vi "Hierarchy To Build Order.vi"(0 "Build Analyzer in":refnum<class "Build Analyzer.lvclass">, 5 "Export Product Names to build":string[](array[string]), 7 "Build Type":T1(ring)) -> (4 "dup Build Analyzer":refnum<class "Build Analyzer.lvclass">, 6 "Ordered Exports":refnum<class "Export.lvclass">[](array[class]), 15 "error out":errorcluster)   [LabVIEW 2017, in "CL_G3_VIComponentBuilder.lvlib" / "Build Analyzer.lvclass"]
doc: "Generates the ordered set of exports to build given the product names of the exports."
uses:
  Build Analyzer.lvclass
  Exports/Exports/Export.lvclass
  Build Analyzer.lvclass/Build Analyzer.ctl
  Exports/Exports/Export.lvclass/Export.ctl
  Exports/Exports/Accessors/Read unique Name.vi
  Exports/Exports/Accessors/Read Product Name.vi
  <userlib>/_Cirrus Logic/LabVIEW Container/Source/Container/Get Child.vi
  <userlib>/_Cirrus Logic/LabVIEW Container/Source/Container/Container.lvclass
panel:
  out "Numeric":i32
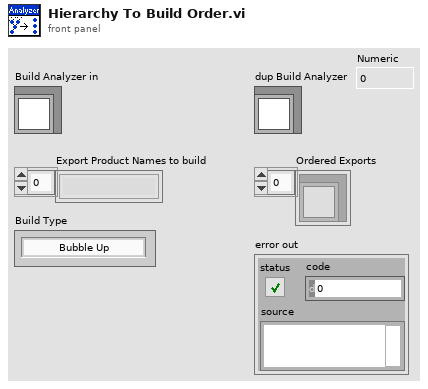
[diagram p1: front panel]
types:
  T1 = enum16{"Bubble Up", "Build Dependencies", "Build Selected Only"}
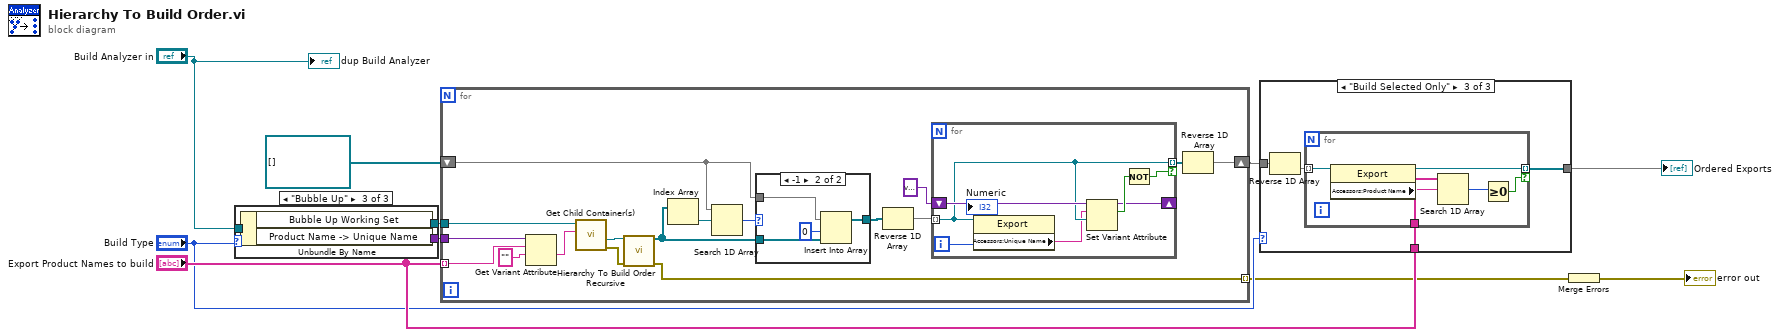
[diagram p0: block diagram]
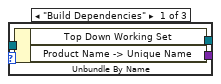
[diagram p2: hidden frame]
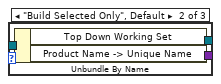
[diagram p3: hidden frame]
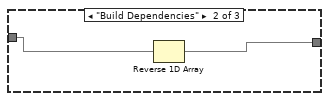
[diagram p5: hidden frame]
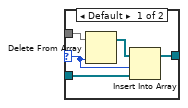
[diagram p6: hidden frame]
diagram:
  n1 = case shown="\"Bubble Up\"" "Build Type" {
    tunnel: [w13 w16 w19] -> w6
    tunnel: [w12 w15 w18] -> w4
    tunnel: "Build Analyzer in" -> [w11 w14 w17]
    frame "Build Dependencies" {
      n2 = Unbundle By Name(w11) -> ("Top Down Working Set"=w13:refnum<data-value>, "Product Name -> Unique Name"=w12:variant)
    }
    frame "Build Selected Only", Default {
      n3 = Unbundle By Name(w14) -> ("Top Down Working Set"=w16:refnum<data-value>, "Product Name -> Unique Name"=w15:variant)
    }
    frame "Bubble Up" {
      n4 = Unbundle By Name(w17) -> ("Bubble Up Working Set"=w19:refnum<data-value>, "Product Name -> Unique Name"=w18:variant)
    }
  }
  n5 = for {
    shift-right: [w20] -> w3
    shift-left: refnum<class "Export.lvclass">[] [] -> [w32]
    tunnel: w6 -> [w24]
    tunnel: "Export Product Names to build" -> [w29] mode=indexing
    tunnel: w4 -> [w30]
    tunnel: [w25] -> w7 mode=indexing
    n6 = Get Variant Attribute(Variant=w30, name=w29, default value (empty Variant)="") -> (value=w27:string)  [unwired: 1 in, 3 out]
    n7 = call-poly <userlib>:"Get Child Container(s).vi"("Container Name"=w27, "Container"=w24) -> ("error out"=w26:errorcluster, "Child Container"=w35:refnum<data-value>)  [unwired: 6 in, 2 out]
    n8 = call "Hierarchy To Build Order Recursive.vi"("Working Set"=w35, "error in (no error)"=w26) -> ("Exports"=w33:refnum<class "Export.lvclass">[], "error out"=w25:errorcluster)  [unwired: 12 in]
    n9 = Index Array(array=w33) -> (element=w34:refnum<class "Export.lvclass">)  [unwired: 1 in]
    n10 = Search 1D Array(1D array=w32, element=w34) -> (index of element=w31:i32)  [unwired: 1 in]
    n11 = case shown="-1" w31 {
      selector: w31 -> [w39 _]
      tunnel: [w37 w45] -> w23
      tunnel: w33 -> [w38 w44]
      tunnel: w32 -> [w41 w43]
      frame Default {
        n12 = Delete From Array(array=w41, index=w39) -> (array with subset deleted=w40:refnum<class "Export.lvclass">[])  [unwired: 1 in, 1 out]
        n13 = Insert Into Array(array=w40, index=w39, new element=w38) -> (w37:refnum<class "Export.lvclass">[])
      }
      frame -1 {
        n14 = Insert Into Array(array=w43, index=0, new element=w44) -> (w45:refnum<class "Export.lvclass">[])
      }
    }
    n15 = Reverse 1D Array(array=w23) -> (reversed array=w22:refnum<class "Export.lvclass">[])
    n16 = for {
      tunnel: w22 -> [w49] mode=indexing
      tunnel: [w49] -> w21 mode=indexing if=w47
      shift-right: [w50] -> _
      shift-left: variant -> [w52]
      i -> [w46]
      # "keep the"
      n17 = property class="Export"(reference=w49) -> ("Accessors:Unique Name"=w48:string)  [unwired: 1 in, 2 out]
      n18 = Set Variant Attribute(Variant=w52, name=w48, value=w49) -> (Variant out=w50:variant, replaced=w51:bool)  [unwired: 1 in, 1 out]
      n19 = Not(x=w51) -> (.not. x?=w47:bool)
      "Numeric" <- w46
    }
    n20 = Reverse 1D Array(array=w21) -> (reversed array=w20:refnum<class "Export.lvclass">[])
  }
  n21 = case shown="\"Build Selected Only\"" "Build Type" {
    tunnel: "Export Product Names to build" -> [_ _ w59]
    tunnel: [w53 w54 w58] -> w10
    tunnel: w3 -> [w53 w55 w57]
    frame "Bubble Up", Default {
    }
    frame "Build Dependencies" {
      n22 = Reverse 1D Array(array=w55) -> (reversed array=w54:refnum<class "Export.lvclass">[])
    }
    frame "Build Selected Only" {
      n23 = Reverse 1D Array(array=w57) -> (reversed array=w56:refnum<class "Export.lvclass">[])
      n24 = for {
        tunnel: w56 -> [w65] mode=indexing
        tunnel: w59 -> [w64]
        tunnel: [w63] -> w58 mode=indexing if=w60
        n25 = property class="Export"(reference=w65) -> (reference out=w63:refnum<class "Export.lvclass">, "Accessors:Product Name"=w61:string)  [unwired: 1 in, 1 out]
        n26 = Search 1D Array(1D array=w64, element=w61) -> (index of element=w62:i32)  [unwired: 1 in]
        n27 = Greater Or Equal To 0?(x=w62) -> (x >= 0?=w60:bool)
      }
    }
  }
  "Ordered Exports" <- w10
  n28 = Merge Errors(w7) -> (→"error out":errorcluster)
  "dup Build Analyzer" <- "Build Analyzer in"
